vi "niTuner Set Freq for SMT.vi"   [LabVIEW 2011]
doc: "This polymorphic VI loads and prepares a scan list of 1 to 720 center frequencies between 9 kHz and 2.6 GHz. When triggered, the PXI-5600 downconverter tunes to these frequencies in succession. Each frequency is associated with a span. The format of the \"spectrum settings\" inputs and outputs is designed to provide a convenient interface with the Spectral Measurements Toolset (SMT).\n\nIf you are working with a single spectrum, you can use the default Set Freq for SMT (spec) instance of this VI. If you are working with multiple spectra, you must use the Set Freq for SMT (Spec Array). To select the Set Freq for SMT (Spec Array) instance, right-click on the Set Freq for SMT icon in your block diagram and click on <B>select type»Set Freq for SMT(Spec Array).vi</B>.\n\nIf you are working with a single spectrum, you can use the default Set Freq for SMT (spec) version of this VI. If you are working with multiple spectra, you must use the Set Freq for SMT (Spec Array). To select the Set Freq for SMT (Spec Array) version, right-click on the Set Freq for SMT icon in your block diagram and click on <B>select type»Set Freq for SMT(Spec Array).vi</B>."
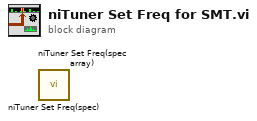
[diagram p0: block diagram]
diagram:
  n1 = call <instrlib>:"niTuner Set Freq(spec).vi"() -> ()  [unwired: 7 in, 5 out]
  n2 = call <instrlib>:"niTuner Set Freq(spec array).vi"() -> ()  [unwired: 7 in, 5 out]
